vi "Stoppani_Bitwise.vi"(6 "Task":T1, 11 "String In":string) -> (0 "Float":dbl, 1 "Int":u32, 2 "Char":bool, 3 "String Out":string, 4 "Array":dbl[](array[numeric]))   [LabVIEW 2022 SP3]
uses:
  Stoppani_Ave_DataType.ctl
panel:
  out "byes":i32
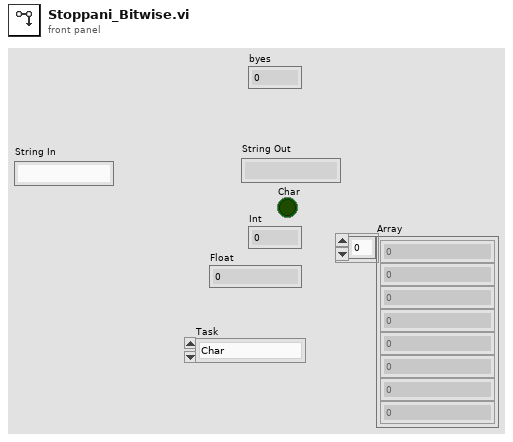
[diagram p1: front panel]
types:
  T1 = typedef "Stoppani_Ave_DataType.ctl" = enum16{"Char", "Byte", "Word", "Int", "Float (SGL)", "Float (DBL)", "Float (DBL Array)"}
  T2 = enum16{"big-endian, network order", "native, host order", "little-endian"}
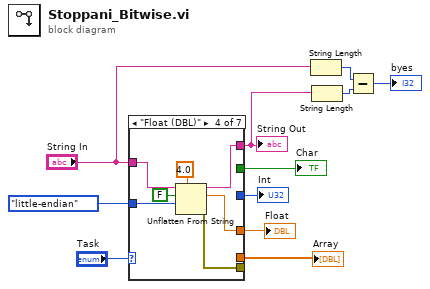
[diagram p0: block diagram]
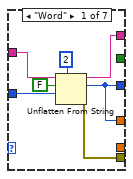
[diagram p2: hidden frame]
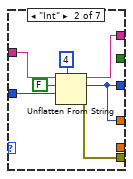
[diagram p3: hidden frame]
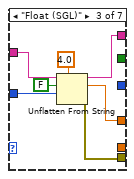
[diagram p4: hidden frame]
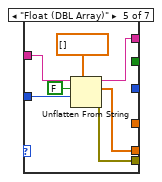
[diagram p5: hidden frame]
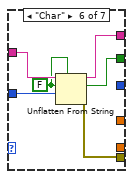
[diagram p6: hidden frame]
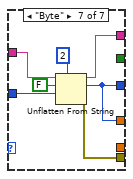
[diagram p7: hidden frame]
diagram:
  n1 = case shown="\"Float (DBL)\"" "Task" {
    tunnel: T2."little-endian" ("byte order (0:big-endian, network order)") -> [w16 w23 w30 w37 w45 w52 w59]
    tunnel: [w15 w22 w29 w36 w44 w51 w58] -> w4
    tunnel: [w13 w20 _ _ _ _ w54] -> w10
    tunnel: "String In" -> [w14 w21 w28 w35 w43 w50 w57]
    tunnel: [w13 w20 w27 w34 _ _ w54] -> w8
    tunnel: [_ _ _ _ _ w48 _] -> w7
    tunnel: [_ _ _ _ w41 _ _] -> w6
    tunnel: [w12 w19 w26 w33 w40 w47 w53] -> _
    frame "Word" {
      n2 = Unflatten From String(type=u16 2 ("count (1)"), binary string=w14, data includes array or string size? (T)=FALSE, byte order (0:big-endian, network order)=w16) -> (rest of the binary string=w15:string, value=w13:u16, error out=w12:errorcluster)  [unwired: 1 in]
    }
    frame "Int" {
      n3 = Unflatten From String(type=u32 4 ("count (1)"), binary string=w21, data includes array or string size? (T)=FALSE, byte order (0:big-endian, network order)=w23) -> (rest of the binary string=w22:string, value=w20:u32, error out=w19:errorcluster)  [unwired: 1 in]
    }
    frame "Float (SGL)" {
      n4 = Unflatten From String(type=sgl 4.0 ("count (1)"), binary string=w28, data includes array or string size? (T)=FALSE, byte order (0:big-endian, network order)=w30) -> (rest of the binary string=w29:string, value=w27:sgl, error out=w26:errorcluster)  [unwired: 1 in]
    }
    frame "Float (DBL)" {
      n5 = Unflatten From String(type=4.0 ("count (1)"), binary string=w35, data includes array or string size? (T)=FALSE, byte order (0:big-endian, network order)=w37) -> (rest of the binary string=w36:string, value=w34:dbl, error out=w33:errorcluster)  [unwired: 1 in]
    }
    frame "Float (DBL Array)" {
      n6 = Unflatten From String(type=dbl[] [], binary string=w43, data includes array or string size? (T)=FALSE, byte order (0:big-endian, network order)=w45) -> (rest of the binary string=w44:string, value=w41:dbl[], error out=w40:errorcluster)  [unwired: 1 in]
    }
    frame "Char" {
      w49 = FALSE ("data includes array or string size? (T)")
      n7 = Unflatten From String(type=w49, binary string=w50, data includes array or string size? (T)=w49, byte order (0:big-endian, network order)=w52) -> (rest of the binary string=w51:string, value=w48:bool, error out=w47:errorcluster)  [unwired: 1 in]
    }
    frame "Byte" {
      n8 = Unflatten From String(type=u8 2 ("count (1)"), binary string=w57, data includes array or string size? (T)=FALSE, byte order (0:big-endian, network order)=w59) -> (rest of the binary string=w58:string, value=w54:u8, error out=w53:errorcluster)  [unwired: 1 in]
    }
  }
  "String Out" <- w4
  "Int" <- w10
  "Float" <- w8
  "Char" <- w7
  "Array" <- w6
  n9 = String Length(string="String In") -> (length=w2:i32)
  n10 = String Length(string=w4) -> (length=w3:i32)
  n11 = Subtract(x=w2, y=w3) -> (x-y=→"byes":i32)
